vi "Approved.vi"(10 "Pass value":dbl, 11 "Average":dbl) -> (2 "Status":bool, 3 "Approved?":string)   [LabVIEW 2025]
doc: "Checks if the Average value is greater than the Pass value and gives a string message of 'approved' if it is greater and a message of 'not approved' if it is not. It also outputs the result in a boolean indicator."
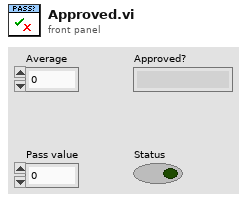
[diagram p1: front panel]
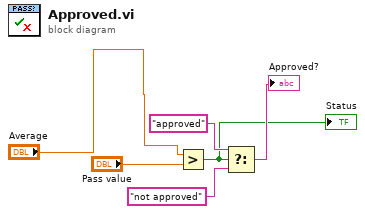
[diagram p0: block diagram]
diagram:
  n1 = Greater?(x="Average", y="Pass value") -> (0:w3:bool)
  "Status" <- w3
  n2 = Select(t="approved" ("format string"), s=w3, f="not approved") -> (s? t:f=→"Approved?":string)
